vi "Filter.vi"(8 "error in (no error)":errorcluster, 10 "Input":sgl[][](array[numeric]), 11 "Speckle Variance Filter in":refnum<class "Speckle Variance Filter.lvclass">) -> (0 "error out":errorcluster, 2 "Output":sgl[][](array[numeric]), 3 "Speckle Variance Filter out":refnum<class "Speckle Variance Filter.lvclass">)   [LabVIEW 2015, in "Speckle Variance Filter.lvclass"]
uses:
  Speckle Variance Filter.lvclass
  Filter.lvclass
  <vilib>/Analysis/NI_AALBase.lvlib
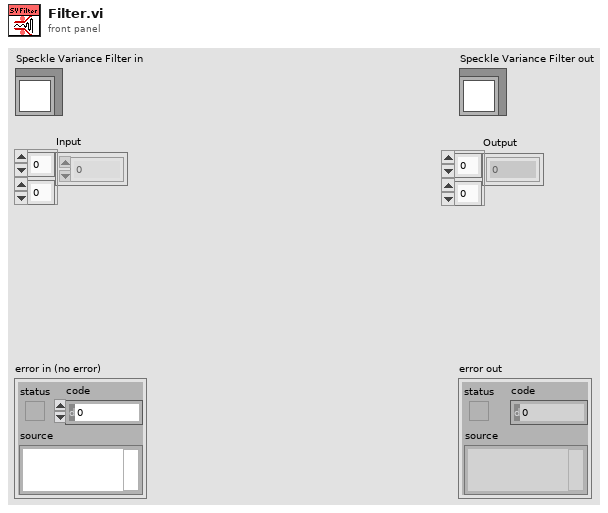
[diagram p1: front panel]
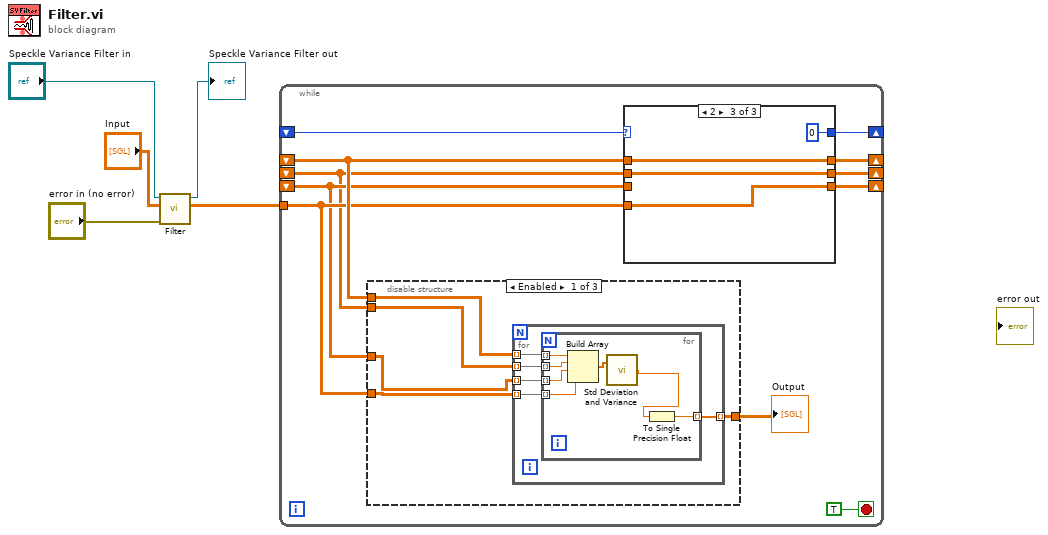
[diagram p0: block diagram]
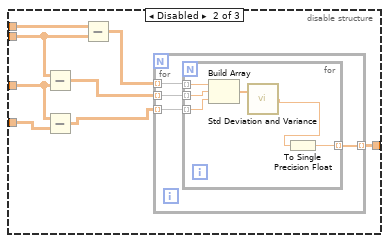
[diagram p2: hidden frame]
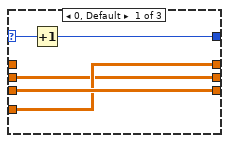
[diagram p4: hidden frame]
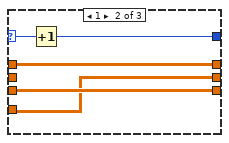
[diagram p5: hidden frame]
diagram:
  n1 = call-parent "Filter.vi"("error in (no error)"="error in (no error)", "Input"="Input", "Filter in"="Speckle Variance Filter in") -> ("Output"=w1:sgl[][], "Filter out"=→"Speckle Variance Filter out":refnum<class "Speckle Variance Filter.lvclass">)  [unwired: 6 in, 1 out]
  n2 = while {
    tunnel: w1 -> [w9]
    shift-right: [w14] -> _
    shift-left: _ -> [w7]
    shift-right: [w13] -> _
    shift-left: _ -> [w10]
    shift-right: [w12] -> _
    shift-left: _ -> [w15]
    shift-right: [w11] -> _
    shift-left: _ -> [w8]
    stop <- TRUE stop-if-true
    n3 = disable-structure shown="Enabled" {
      disable-tunnel: w10 -> [w20 w41 _]
      disable-tunnel: w9 -> [w17 w40 _]
      disable-tunnel: w8 -> [w18 w39 _]
      disable-tunnel: w7 -> [w19 w38 _]
      disable-tunnel: [w21 w37 _] -> w6
      frame Enabled {
        n4 = for {
          tunnel: w20 -> [w24] mode=indexing
          tunnel: w19 -> [w25] mode=indexing
          tunnel: w18 -> [w26] mode=indexing
          tunnel: [w23] -> w21 mode=indexing
          tunnel: w17 -> [w22] mode=indexing
          n5 = for {
            tunnel: w26 -> [w31] mode=indexing
            tunnel: w25 -> [w32] mode=indexing
            tunnel: w24 -> [w33] mode=indexing
            tunnel: [w29] -> w23 mode=indexing
            tunnel: w22 -> [w27] mode=indexing
            n6 = Build Array(w33, w32, w31, w27) -> (w30:sgl[])
            n7 = call <vilib>:"Std Deviation and Variance.vi"("X"=w30) -> ("standard deviation"=w28:dbl)  [unwired: 1 in, 2 out]
            n8 = To Single Precision Float(number=w28) -> (single precision float=w29:sgl)
          }
        }
      }
      frame Disabled {
        n9 = Subtract(x=w38, y=w39) -> (x-y=w35:sgl[][])
        n10 = Subtract(x=w39, y=w40) -> (x-y=w36:sgl[][])
        n11 = Subtract(x=w41, y=w38) -> (x-y=w34:sgl[][])
        n12 = for {
          tunnel: w34 -> [w43] mode=indexing
          tunnel: w35 -> [w44] mode=indexing
          tunnel: w36 -> [w45] mode=indexing
          tunnel: [w42] -> w37 mode=indexing
          n13 = for {
            tunnel: w45 -> [w49] mode=indexing
            tunnel: w44 -> [w50] mode=indexing
            tunnel: w43 -> [w51] mode=indexing
            tunnel: [w47] -> w42 mode=indexing
            n14 = Build Array(w51, w50, w49) -> (w48:sgl[])
            n15 = call <vilib>:"Std Deviation and Variance.vi"("X"=w48) -> ("standard deviation"=w46:dbl)  [unwired: 1 in, 2 out]
            n16 = To Single Precision Float(number=w46) -> (single precision float=w47:sgl)
          }
        }
      }
      frame Disabled {
      }
    }
    "Output" <- w6
    n17 = case shown="2" w15 {
      selector: w15 -> [w56 w61 _]
      tunnel: [w52 w58 w63] -> w14
      tunnel: w9 -> [w53 w58 w64]
      tunnel: w7 -> [w52 _ w63]
      tunnel: [w53 w57 w62] -> w13
      tunnel: w10 -> [_ w57 w62]
      tunnel: [w55 w59 0] -> w12
      tunnel: w8 -> [w54 w60 _]
      tunnel: [w54 w60 w64] -> w11
      frame 0, Default {
        n18 = Increment(x=w56) -> (x+1=w55:i32)
      }
      frame 1 {
        n19 = Increment(x=w61) -> (x+1=w59:i32)
      }
      frame 2 {
      }
    }
  }
